vi "nanocal-frontend-tcplink-client-LV19.vi"() -> ()   [LabVIEW 2019]
doc: "Demonstrates how to open a connection to an TCP server, read the data being sent, and display the data on a chart. This VI is designed to stop if the TCP connection is terminated."
uses:
  publisher action.ctl
  icicle.ctl
panel:
  in  "Tab Control":enum32{"Page 1", "Page 2"}(tab)
  in  "Stop":bool
  in  "address":string="146.201.231.45"
  in  "port":u16=6340
  in  "wait (ms)":u32=100
  in  "timeout ms (25000)":i32=1000
  out "nanocal data array OUT":T1[](array[typedef])
  # "nanocal tcplink --- client"
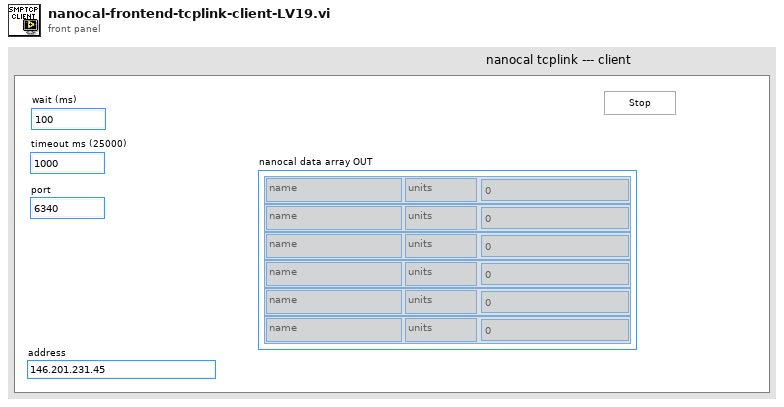
[diagram p1: front panel]
types:
  T1 = typedef "icicle.ctl" = cluster{"name":string, "units":string, "data":dbl}
  T2 = typedef "publisher action.ctl" = enum16{"set", "get", "init", "check"}
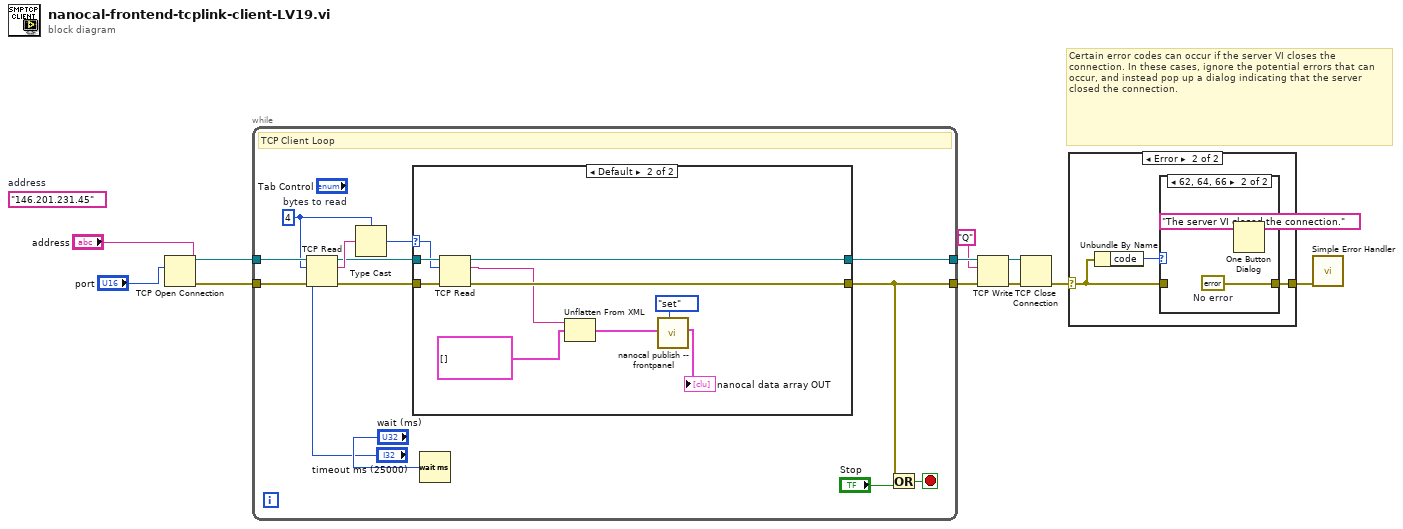
[diagram p0: block diagram]
diagram:
  (unwired) "146.201.231.45"  # address
  # "Certain error codes can occur if the server VI closes the connection. In these cases, ignore the potential errors that can occur, and instead pop up a dialog indicating that the server closed the connection."
  n1 = TCP Open Connection(address="address", remote port or service name="port") -> (connection ID=w11:refnum<k5>, error out=w10:errorcluster)  [unwired: 3 in]
  n2 = while {
    tunnel: w10 -> [w20]
    tunnel: w11 -> [w21]
    tunnel: [w15] -> w8
    tunnel: [w14] -> w6
    stop <- w17 stop-if-true
    w19 = 4  # bytes to read
    # "TCP Client Loop"
    n3 = TCP Read(connection ID=w21, bytes to read=w19, error in (no error)=w20, 9:"timeout ms (25000)") -> (connection ID out=w23:refnum<k5>, data out=w24:string, error out=w22:errorcluster)  [unwired: 1 in]
    n4 = Type Cast(type=w19, x=w24) -> (*(type *) &x=w13:i32)
    n5 = case shown="Default" w13 {
      selector: w13 -> [_ w32]
      tunnel: w23 -> [w26 w36]
      tunnel: w22 -> [w25 w35]
      tunnel: [w26 w34] -> w15
      tunnel: [w25 w33] -> w14
      frame ..0 {
        # "The server has not written any data"
      }
      frame Default {
        n6 = TCP Read(connection ID=w36, bytes to read=w32, error in (no error)=w35) -> (connection ID out=w34:refnum<k5>, data out=w31:string, error out=w33:errorcluster)  [unwired: 2 in]
        n7 = Unflatten From XML(xml string=w31, type=T1[] []) -> (value=w28:T1[])  [unwired: 1 in, 1 out]
        n8 = call "nanocal publish -- frontpanel.vi"("publisher action"=publisher_action."set", "nanocal data array IN"=w28) -> ("nanocal data array OUT"=→"nanocal data array OUT":T1[])  [unwired: 9 in]
      }
    }
    n9 = Wait (ms)(milliseconds to wait="wait (ms)") -> ()  [unwired: 1 out]
    n10 = Or(x=w14, y="Stop") -> (x .or. y?=w17:bool)
  }
  n11 = TCP Write(connection ID=w8, data in="Q", error in (no error)=w6) -> (connection ID out=w9:refnum<k5>, error out=w7:errorcluster)  [unwired: 2 out]
  n12 = TCP Close Connection(connection ID=w9, error in (no error)=w7) -> (error out=w4:errorcluster)  [unwired: 1 in, 1 out]
  n13 = case shown="Error" w4 {
    selector: w4 -> [w37 w39]
    tunnel: [w37 w38] -> w3
    frame No Error {
    }
    frame Error {
      n14 = Unbundle By Name(w39) -> ("code"=w40:i32)
      n15 = case shown="62, 64, 66" w40 {
        tunnel: w39 -> [w41 _]
        tunnel: [w41 w43] -> w38
        frame Default {
        }
        frame 62, 64, 66 {
          w43 = errorcluster {"status"=FALSE, "code"=0, "source"=""}  # No error
          n16 = One Button Dialog(message="The server VI closed the connection." ("Server Closed")) -> ()  [unwired: 1 in, 1 out]
        }
      }
    }
  }
  n17 = call <vilib>:"Simple Error Handler.vi"("error in (no error)"=w3) -> ()  [unwired: 4 in, 5 out]
